vi "ExecPratAula02.vi"() -> ()   [LabVIEW 2020]
panel:
  in  "Numeric 5":fxp<+/-,64,32>
  in  "Numeric":fxp<+/-,64,32>
  out "Slide":u8(slide) scale=0.0..200.0
  in  "Numeric 3":fxp<+/-,64,32>
  in  "Numeric 4":fxp<+/-,64,32>
  out "(i)":i32
  in  "Numeric 2":fxp<+/-,64,32>
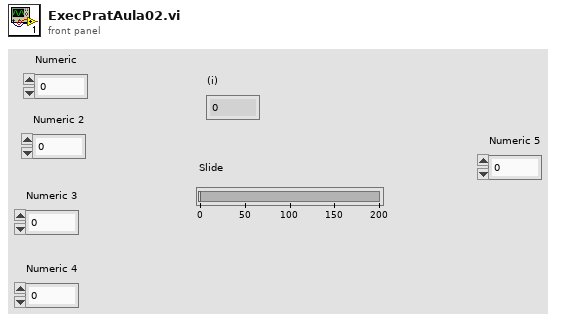
[diagram p1: front panel]
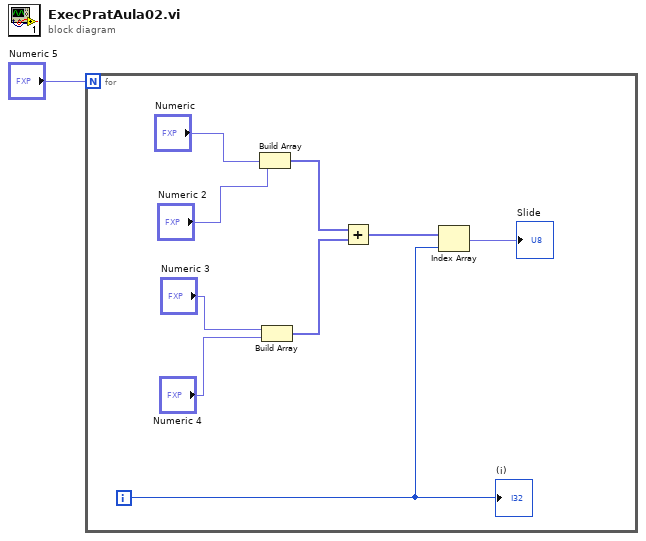
[diagram p0: block diagram]
diagram:
  n1 = for {
    N: "Numeric 5" -> [_]
    i -> [w4]
    n2 = Build Array("Numeric", "Numeric 2") -> (w7:fxp<+/-,64,32>[])
    n3 = Build Array("Numeric 3", "Numeric 4") -> (w6:fxp<+/-,64,32>[])
    n4 = Add(x=w7, y=w6) -> (x+y=w5:fxp<+/-,64,33>[])
    n5 = Index Array(array=w5, index=w4) -> (element=→"Slide":fxp<+/-,64,33>)
    "(i)" <- w4
  }
